vi "read_NI - scan.vi"() -> (0 "all_pds":dbl[](array[numeric]), 1 "-pd3/pd1":dbl, 2 "pd3/pd1":dbl, 4 "error out":errorcluster)   [LabVIEW 2024]
uses:
  <vilib>/Analysis/NI_AALBase.lvlib
panel:
  out "dt":u32
  out "pd2/pd1":dbl
  out "ch2-sd":dbl format="%^#_6g"
  out "ch2-avg":dbl format="%^#_6g"
  out "ch1-sd":dbl format="%^#_6g"
  out "ch1-avg":dbl format="%^#_6g"
  out "ch0-sd":dbl format="%^#_6g"
  out "ch0-avg":dbl format="%^#_6g"
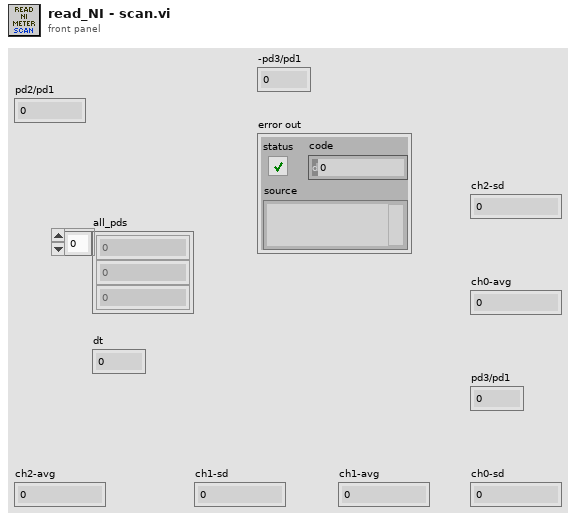
[diagram p1: front panel]
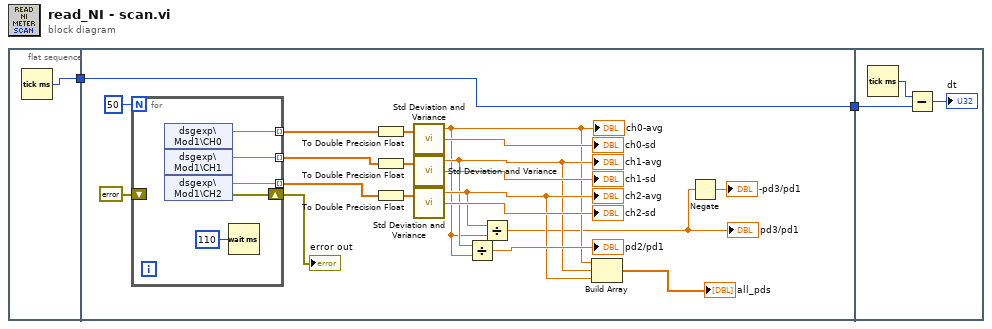
[diagram p0: block diagram]
diagram:
  n1 = flat-sequence {
    tunnel: [w3] -> w2
    tunnel: w2 -> [w4]
    tunnel: [w4] -> w1
    tunnel: w1 -> [w32]
    frame #0 {
      n2 = Tick Count (ms)() -> (millisecond timer value=w3:u32)
    }
    frame #1 {
      n3 = for {
        N: 50 -> [_]
        tunnel: [w30] -> w9 mode=indexing
        tunnel: [w29] -> w8 mode=indexing
        tunnel: [w28] -> w7 mode=indexing
        shift-right: [w24] -> w6
        shift-left: errorcluster {"status"=FALSE, "code"=0, "source"=""} ("error IO") -> [_]
        n4 = shared-variable "dsgexp\\Mod1\\CH0"() -> (w30:dbl, error out=w26:errorcluster)  [unwired: 1 in]
        n5 = shared-variable "dsgexp\\Mod1\\CH1"(error in=w26) -> (w29:dbl, error out=w25:errorcluster)
        n6 = shared-variable "dsgexp\\Mod1\\CH2"(error in=w25) -> (w28:dbl, error out=w24:errorcluster)
        n7 = Wait (ms)(milliseconds to wait=u32 110) -> ()  [unwired: 1 out]
      }
      "error out" <- w6
      n8 = To Double Precision Float(number=w9) -> (double precision float=w14:dbl[])
      n9 = To Double Precision Float(number=w8) -> (double precision float=w13:dbl[])
      n10 = To Double Precision Float(number=w7) -> (double precision float=w15:dbl[])
      n11 = call <vilib>:"Std Deviation and Variance.vi"("X"=w14) -> ("mean"=w16:dbl, "standard deviation"=→"ch0-sd":dbl)  [unwired: 1 in, 1 out]
      "ch0-avg" <- w16
      n12 = call <vilib>:"Std Deviation and Variance.vi"("X"=w13) -> ("mean"=w18:dbl, "standard deviation"=→"ch1-sd":dbl)  [unwired: 1 in, 1 out]
      "ch1-avg" <- w18
      n13 = call <vilib>:"Std Deviation and Variance.vi"("X"=w15) -> ("mean"=w19:dbl, "standard deviation"=→"ch2-sd":dbl)  [unwired: 1 in, 1 out]
      "ch2-avg" <- w19
      n14 = Divide(x=w18, y=w16) -> (x/y=→"pd2/pd1":dbl)
      n15 = Divide(x=w19, y=w16) -> (x/y=w11:dbl)
      "pd3/pd1" <- w11
      n16 = Build Array(w16, w18, w19) -> (→"all_pds":dbl[])
      n17 = Negate(x=w11) -> (-x=→"-pd3/pd1":dbl)
    }
    frame #2 {
      n18 = Tick Count (ms)() -> (millisecond timer value=w33:u32)
      n19 = Subtract(x=w33, y=w32) -> (x-y=→"dt":u32)
    }
  }
